vi "Vbg_sweep_for_different_configs.vi"(1 "step":dbl=0.35, 2 "Comments":string="SA02701K.20130901\n\n7 configs, 3 IV at each config (including 2 terminal 27/28)\nVbg sweep -7V to 7V in .0.35 V step\n\nTriangle 1 mVac+250mVdc\n", 3 "2 Terminal Current Measurements":T2(array[cluster])=[{"26"=["NC"], "27"=["NC"], "28"=["y7"], "1"=["y8"], "2"=["y4"], "3"=["y3"], "4"=["y5"], "5"=["y1"]}, {"26"=["NC"], "27"=["NC"], "28"=["y7"], "1"=["y8"], "2"=["y4"], "3"=["y3"], "4"=["y5"], "5"=["y1"]}, {"26"=["NC"], "27"=["NC"], "28"=["y7"], "1"=["y8"], "2"=["y4"], "3"=["y3"], "4"=["y5"], "5"=["y1"]}, {"26"=["NC"], "27"=["NC"], "28"=["y7"], "1"=["y8"], "2"=["y4"], "3"=["y3"], "4"=["y5"], "5"=["y1"]}, {"26"=["NC"], "27"=["NC"], "28"=["y7"], "1"=["y8"], "2"=["y4"], "3"=["y3"], "4"=["y5"], "5"=["y1"]}, {"26"=["NC"], "27"=["NC"], "28"=["y7"], "1"=["y8"], "2"=["y4"], "3"=["y3"], "4"=["y5"], "5"=["y1"]}, {"26"=["NC"], "27"=["NC"], "28"=["y7"], "1"=["y8"], "2"=["y4"], "3"=["y3"], "4"=["y5"], "5"=["y1"]}], 5 "end":dbl=7.0, 7 "start":dbl=-7.0) -> ()   [LabVIEW 2013]
uses:
  <userlib>/LevyLab/PPMS_VIs/Lockin-4461_MultiChannel - IV 3.0 globals.vi
panel:
  in  "OK Button":bool
  in  "Enum":enum16{"linear", "power"}(ring)
  in  "Experiment folder name":string="IV_Vbg_sweep_7configs"
  in  "< T (only valid in B sweep)":dbl=0.055
  in  "(field or temp) end":dbl
  in  "(field or temp) start":dbl
  in  "(field or temp) step":dbl
  in  "Temp / Field":bool=TRUE
  in  "Disable Auto Adjust?":bool=TRUE
  in  "Backgate sweep?":bool=TRUE
  in  "Increase bias if insulating":dbl=0.0005 format="%#_6p"
  in  "Max current":dbl=5e-08 format="%#_6p"
  in  "OSC Configuration":T1(array[cluster])=[{"Signal Type"=enum."Triangle Wave", "DC"=0.00025, "Amplitude"=0.0005, "frequency"=0.1, "Phase"=0.0}, {"Signal Type"=enum."Sine Wave", "DC"=0.0, "Amplitude"=0.0, "frequency"=1.0, "Phase"=0.0}, {"Signal Type"=enum."Sine Wave", "DC"=0.0, "Amplitude"=0.0, "frequency"=1.0, "Phase"=0.0}, {"Signal Type"=enum."Sine Wave", "DC"=0.0, "Amplitude"=0.0, "frequency"=1.0, "Phase"=0.0}] {"frequency" format="%0.2p"; "Amplitude" format="%0.2p"; "DC" min=-0.99 max=0.99 format="%.2p"}
  in  "Wait after backgate":u32=12000
  in  "# IV curves":i32=3
  in  "Wait time after switching":u32=10000
  in  "Tab Control":enum32{"2 Terminal Current Measurements"}(tab)
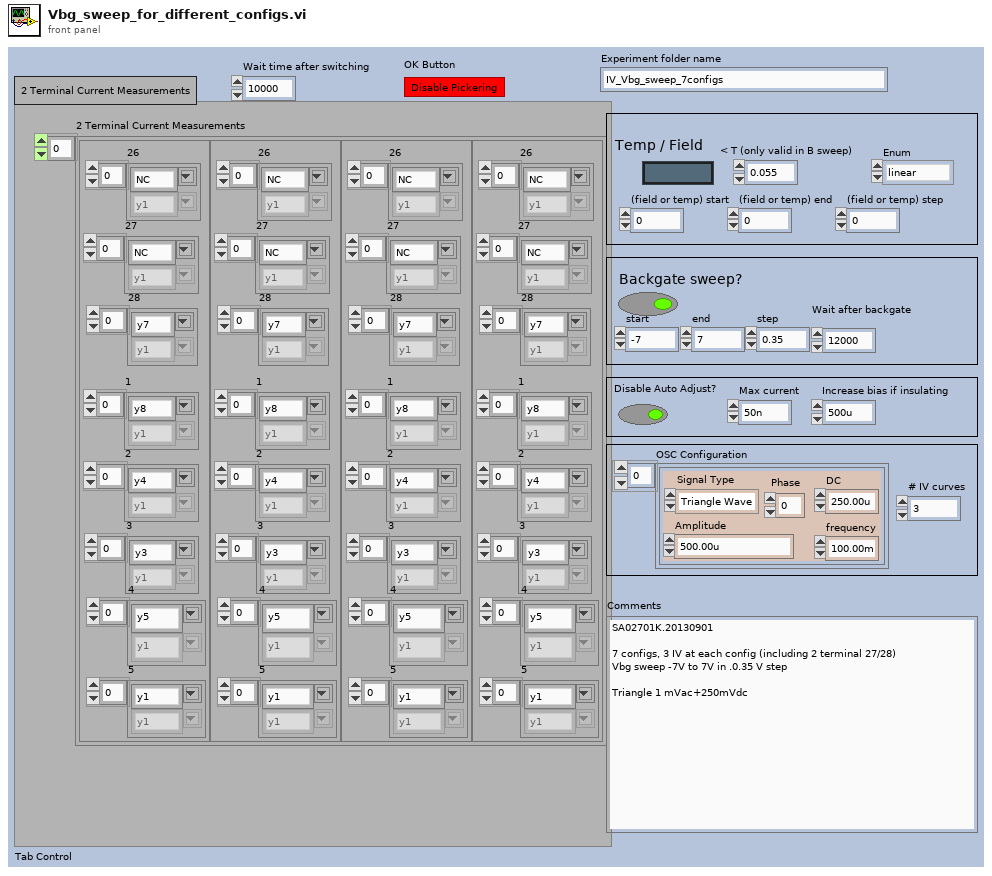
[diagram p1: front panel]
types:
  T1 = cluster{"Signal Type":enum16{"Sine Wave", "Triangle Wave", "Square Wave", "Sawtooth Wave"}, "DC":dbl, "Amplitude":dbl, "frequency":dbl, "Phase":dbl}[]
  T2 = cluster{"26":string[], "27":string[], "28":string[], "1":string[], "2":string[], "3":string[], "4":string[], "5":string[]}[]
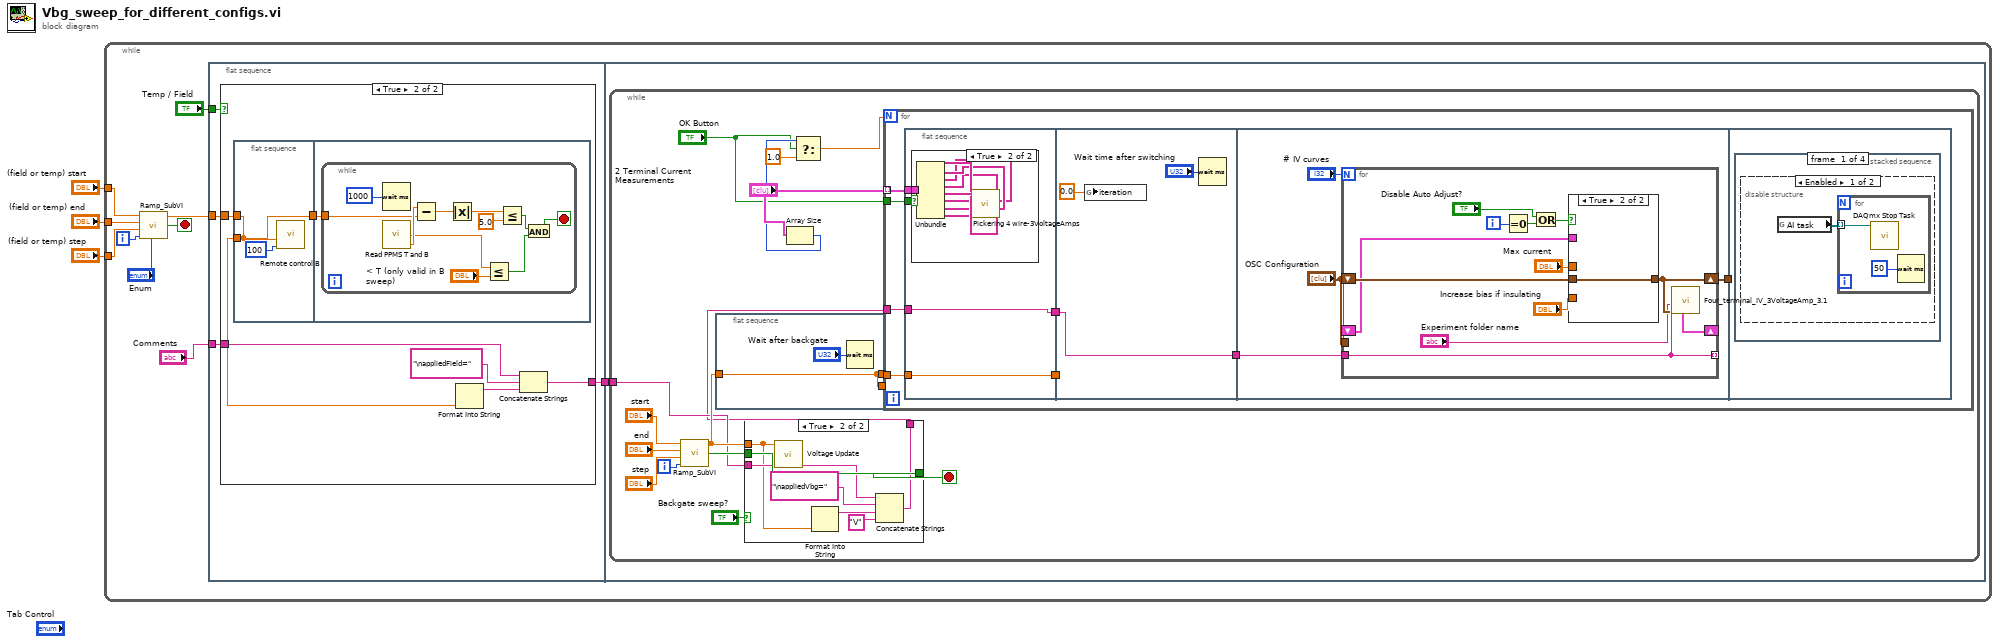
[diagram p0: block diagram]
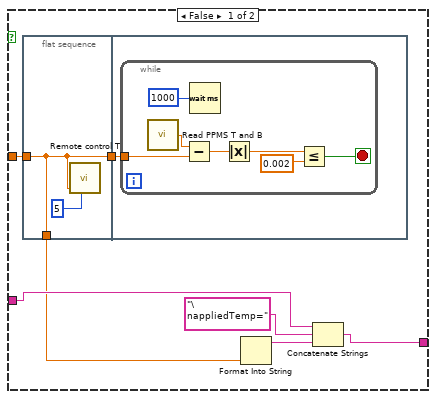
[diagram p2: hidden frame]
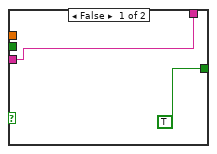
[diagram p3: hidden frame]
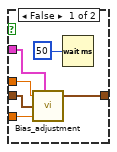
[diagram p5: hidden frame]
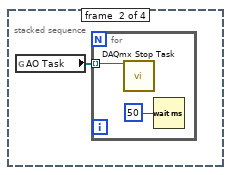
[diagram p7: hidden frame]
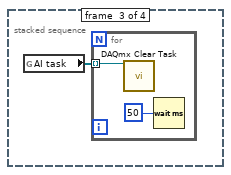
[diagram p8: hidden frame]
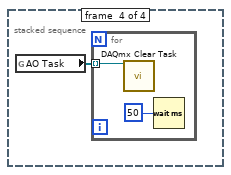
[diagram p9: hidden frame]
diagram:
  n1 = while {
    tunnel: "(field or temp) step" -> [w10]
    tunnel: "(field or temp) start" -> [w9]
    tunnel: "(field or temp) end" -> [w8]
    i -> [w13]
    stop <- w12 stop-if-true
    n2 = call <userlib>:"Ramp_SubVI.vi"("Enum"="Enum", "index"=w13, "step"=w10, "end"=w8, "start"=w9) -> ("Stop?"=w12:bool, "Numeric"=w11:dbl)
    n3 = flat-sequence {
      tunnel: w11 -> [w17]
      tunnel: "Temp / Field" -> [w16]
      tunnel: "Comments" -> [w15]
      tunnel: [w14] -> w5
      tunnel: w5 -> [w56]
      frame #0 {
        n4 = case shown="True" w16 {
          tunnel: w17 -> [w23 w40]
          tunnel: w15 -> [w20 w36]
          tunnel: [w19 w35] -> w14
          frame False {
            n5 = flat-sequence {
              tunnel: w23 -> [w25]
              tunnel: [w25] -> w24
              tunnel: [w25] -> w18
              tunnel: w24 -> [w27]
              frame #0 {
                n6 = call <vilib>:"Remote control T.vi"("Temperature (K)"=w25, "Rate (K/min)"=5 ("Rate (Oe/s)")) -> ()  [unwired: 4 in]
              }
              frame #1 {
                n7 = while {
                  tunnel: w27 -> [w31]
                  stop <- w28 stop-if-true
                  n8 = call "Read PPMS T and B.vi"() -> ("Temperature"=w29:dbl)  [unwired: 3 in, 2 out]
                  n9 = Subtract(x=w29, y=w31) -> (x-y=w34:dbl)
                  n10 = Wait (ms)(milliseconds to wait=u32 1000) -> ()  [unwired: 1 out]
                  n11 = Absolute Value(x=w34) -> (abs(x)=w33:dbl)
                  n12 = Less Or Equal?(x=w33, y=0.002) -> (x <= y?=w28:bool)
                }
              }
            }
            n13 = Format Into String(w18) -> (resulting string=w21:string)  [unwired: 3 in, 1 out]
            n14 = Concatenate Strings(w20, "\nappliedTemp=" ("string"), w21) -> (w19:string)
          }
          frame True {
            n15 = flat-sequence {
              tunnel: w40 -> [w42]
              tunnel: [w42] -> w41
              tunnel: [w42] -> w37
              tunnel: w41 -> [w44]
              frame #0 {
                n16 = call "Remote control B.vi"("Rate (Oe/s)"=100, "Field (Oe)"=w42) -> ()  [unwired: 7 in, 1 out]
              }
              frame #1 {
                n17 = while {
                  tunnel: w44 -> [w51]
                  stop <- w45 stop-if-true
                  n18 = Wait (ms)(milliseconds to wait=u32 1000) -> ()  [unwired: 1 out]
                  n19 = call "Read PPMS T and B.vi"() -> ("Field"=w55:dbl, "Temperature"=w49:dbl)  [unwired: 3 in, 1 out]
                  n20 = Subtract(x=w55, y=w51) -> (x-y=w54:dbl)
                  n21 = Absolute Value(x=w54) -> (abs(x)=w53:dbl)
                  n22 = Less Or Equal?(x=w49, y="< T (only valid in B sweep)") -> (x <= y?=w47:bool)
                  n23 = Less Or Equal?(x=w53, y=5.0) -> (x <= y?=w46:bool)
                  n24 = And(x=w46, y=w47) -> (x .and. y?=w45:bool)
                }
              }
            }
            n25 = Format Into String(w37) -> (resulting string=w38:string)  [unwired: 3 in, 1 out]
            n26 = Concatenate Strings(w36, "\nappliedField=" ("string"), w38) -> (w35:string)
          }
        }
      }
      frame #1 {
        n27 = while {
          tunnel: w56 -> [w63]
          i -> [w65]
          stop <- w70 stop-if-true
          n28 = call <userlib>:"Ramp_SubVI.vi"("index"=w65, "step"="step", "end"="end", "start"="start") -> ("Stop?"=w66:bool, "Numeric"=w64:dbl)  [unwired: 1 in]
          n29 = flat-sequence {
            tunnel: w64 -> [w83]
            tunnel: [w83] -> _
            tunnel: [w83] -> w72
            frame #0 {
              n30 = Wait (ms)(milliseconds to wait="Wait after backgate") -> ()  [unwired: 1 out]
            }
          }
          n31 = case shown="True" "Backgate sweep?" {
            tunnel: w66 -> [_ w81]
            tunnel: [TRUE ("Stop?") w81] -> w70
            tunnel: w64 -> [_ w76]
            tunnel: w63 -> [w73 w77]
            tunnel: [w73 w75] -> w62
            frame False {
            }
            frame True {
              n32 = call "Voltage Update.vi"("Voltage Output"=w76) -> ()  [unwired: 7 in, 1 out]
              n33 = Format Into String(w76) -> (resulting string=w79:string)  [unwired: 3 in, 1 out]
              n34 = Concatenate Strings(w77, "\nappliedVbg=" ("string"), w79, "V" ("string")) -> (w75:string)
            }
          }
          n35 = Array Size(array="2 Terminal Current Measurements") -> (size(s)=w59:i32)
          n36 = Select(t=w59, s="OK Button", f=1.0) -> (s? t:f=w58:dbl)
          n37 = for {
            N: w58 -> [_]
            tunnel: "2 Terminal Current Measurements" -> [w91] mode=indexing
            tunnel: w72 -> [w88]
            tunnel: w62 -> [w85]
            tunnel: "OK Button" -> [w84]
            n38 = flat-sequence {
              tunnel: [w93] -> w90
              tunnel: w91 -> [w95]
              tunnel: w88 -> [w94]
              tunnel: [w94] -> w87
              tunnel: w85 -> [w93]
              tunnel: w84 -> [w92]
              tunnel: w90 -> [w105]
              tunnel: [w105] -> w89
              tunnel: w87 -> [_]
              tunnel: w89 -> [w110]
              tunnel: [w108] -> w86
              tunnel: w86 -> [_]
              frame #0 {
                n39 = case shown="True" w92 {
                  tunnel: w95 -> [_ w104]
                  frame False {
                  }
                  frame True {
                    n40 = Unbundle(w104) -> ("26"=w102:string[], "27"=w101:string[], "28"=w100:string[], "1"=w99:string[], "2"=w103:string[], "3"=w98:string[], "4"=w97:string[], "5"=w96:string[])
                    n41 = call <userlib>:"Pickering 4 wire-3VoltageAmps.vi"("26"=w102, "27"=w101, "28"=w100, "1"=w99, "5"=w96, "4"=w97, "3"=w98, "2"=w103) -> ()  [unwired: 4 in]
                  }
                }
              }
              frame #1 {
                n42 = global write "Lockin-4461_MultiChannel - IV 3.0 globals.vi" "iteration"(0.0 ("iteration")) -> ()
                n43 = Wait (ms)(milliseconds to wait="Wait time after switching") -> ()  [unwired: 1 out]
              }
              frame #2 {
                n44 = for {
                  N: "# IV curves" -> [_]
                  tunnel: w110 -> [w115]
                  tunnel: [w115] -> _ mode=indexing
                  shift-right: [w114] -> w108
                  shift-left: "OSC Configuration" -> [w123]
                  shift-right: [w113] -> _
                  shift-left: _ -> [w120]
                  tunnel: "OSC Configuration" -> [_]
                  i -> [w119]
                  n45 = Equal To 0?(x=w119) -> (x = 0?=w118:bool)
                  n46 = Or(x="Disable Auto Adjust?", y=w118) -> (x .or. y?=w117:bool)
                  n47 = case shown="True" w117 {
                    tunnel: w123 -> [w129 w130]
                    tunnel: "Max current" -> [w128 _]
                    tunnel: "Increase bias if insulating" -> [w127 _]
                    tunnel: [w126 w130] -> w114
                    tunnel: w120 -> [w125 _]
                    frame False {
                      n48 = call "Bias_adjustment.vi"("Base current"=w128, "Two terminal IV"=w125, "OSC Configuration"=w129, "Delta"=w127) -> ("OSC Configuration 2"=w126:T1)  [unwired: 3 in]
                      n49 = Wait (ms)(milliseconds to wait=u32 50) -> ()  [unwired: 1 out]
                    }
                    frame True {
                    }
                  }
                  n50 = call <userlib>:"Four_terminal_IV_3VoltageAmp_3.1.vi"("OSC Configuration"=w114, "Experiment folder name"="Experiment folder name", "Comments"=w115) -> ("Two terminal IV"=w113:cluster{dbl[], dbl[]})  [unwired: 2 in, 4 out]
                }
              }
              frame #3 {
                n51 = stacked-sequence {
                  frame #0 {
                    n52 = disable-structure shown="Enabled" {
                      frame Enabled {
                        n53 = global read "Lockin-4461_MultiChannel - IV 3.0 globals.vi" "AI task"() -> (w131:refnum<k21>[])
                        n54 = for {
                          tunnel: w131 -> [w133] mode=indexing
                          n55 = call <vilib>:"DAQmx Stop Task.vi"("task/channels in"=w133) -> ()  [unwired: 13 in, 2 out]
                          n56 = Wait (ms)(milliseconds to wait=u32 50) -> ()  [unwired: 1 out]
                        }
                      }
                      frame Disabled {
                      }
                    }
                  }
                  frame #1 {
                    n57 = global read "Lockin-4461_MultiChannel - IV 3.0 globals.vi" "AO Task"() -> (w134:refnum<k21>[])
                    n58 = for {
                      tunnel: w134 -> [w136] mode=indexing
                      n59 = call <vilib>:"DAQmx Stop Task.vi"("task/channels in"=w136) -> ()  [unwired: 13 in, 2 out]
                      n60 = Wait (ms)(milliseconds to wait=u32 50) -> ()  [unwired: 1 out]
                    }
                  }
                  frame #2 {
                    n61 = global read "Lockin-4461_MultiChannel - IV 3.0 globals.vi" "AI task"() -> (w137:refnum<k21>[])
                    n62 = for {
                      tunnel: w137 -> [w139] mode=indexing
                      n63 = call <vilib>:"DAQmx Clear Task.vi"("task in"=w139) -> ()  [unwired: 14 in, 1 out]
                      n64 = Wait (ms)(milliseconds to wait=u32 50) -> ()  [unwired: 1 out]
                    }
                  }
                  frame #3 {
                    n65 = global read "Lockin-4461_MultiChannel - IV 3.0 globals.vi" "AO Task"() -> (w140:refnum<k21>[])
                    n66 = for {
                      tunnel: w140 -> [w142] mode=indexing
                      n67 = call <vilib>:"DAQmx Clear Task.vi"("task in"=w142) -> ()  [unwired: 14 in, 1 out]
                      n68 = Wait (ms)(milliseconds to wait=u32 50) -> ()  [unwired: 1 out]
                    }
                  }
                }
              }
            }
          }
        }
      }
    }
  }
